vi "TALOS Root path.vi"(8 "error in (no error)":errorcluster) -> (0 "error out":errorcluster, 3 "TALOS Root Path":path)   [LabVIEW 2026, in "TALOS.lvlib"]
doc: "This VI gives the path to the root of the folder tree."
uses:
  TALOS.lvlib
  Global Memory.vi
  <vilib>/Utility/LVLibp/NI_PackedLibraryUtility.lvlib
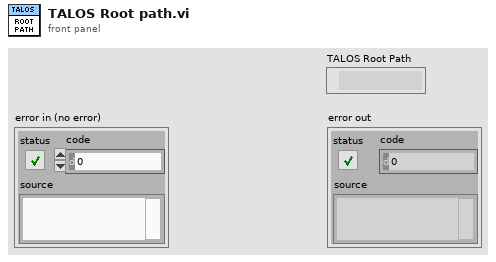
[diagram p1: front panel]
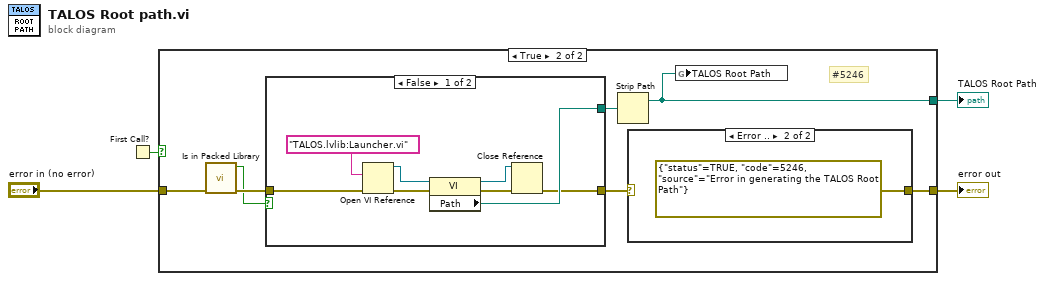
[diagram p0: block diagram]
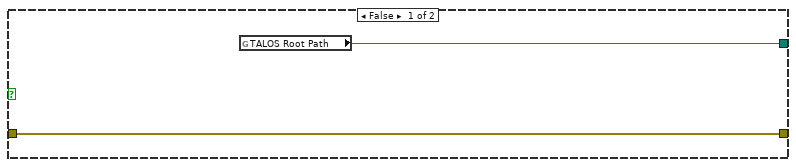
[diagram p2: hidden frame]
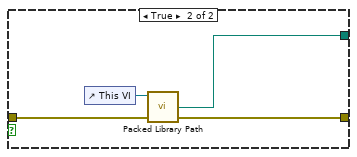
[diagram p4: hidden frame]
diagram:
  n1 = First Call?() -> (First Call?: T/F=w1:bool)
  n2 = case shown="True" w1 {
    tunnel: [w5 w12] -> w4
    tunnel: [w6 w7] -> w3
    tunnel: "error in (no error)" -> [w6 w11]
    frame False {
      n3 = global read "Global Memory.vi" "TALOS Root Path"() -> (w5:path)
    }
    frame True {
      # "#5246"
      n4 = call "Is in Packed Library.vi"("error in (no error)"=w11) -> ("error out"=w10:errorcluster, "Is In Packed Library"=w9:bool)  [unwired: 9 in]
      n5 = case shown="False" w9 {
        tunnel: w10 -> [w23 w27]
        tunnel: [w16 w24] -> w8
        tunnel: [w17 w25] -> w13
        frame False {
          n6 = Open VI Reference(vi path="TALOS.lvlib:Launcher.vi" ("string"), error in (no error)=w23) -> (vi reference=w20:refnum<vi>, error out=w21:errorcluster)  [unwired: 4 in]
          n7 = property class="VI"(reference=w20, error in=w21) -> (reference out=w18:refnum<vi>, error out=w19:errorcluster, "Path"=w17:path)
          n8 = Close Reference(reference=w18, error in (no error)=w19) -> (error out=w16:errorcluster)
        }
        frame True {
          n9 = control-ref of="This VI"() -> (w26:refnum<vi>)
          n10 = call <vilib>:"Packed Library Path.vi"("error in (no error)"=w27, "vi reference"=w26) -> ("error out"=w24:errorcluster, "packed library path"=w25:path)  [unwired: 1 in, 1 out]
        }
      }
      n11 = Strip Path(path=w13) -> (stripped path=w12:path)  [unwired: 1 out]
      n12 = case shown="Error .." w8 {
        selector: w8 -> [w14 _]
        tunnel: [w14 errorcluster {"status"=TRUE, "code"=5246, "source"="Error in generating the TALOS Root Path"} ("error IO")] -> w7
        frame No Error {
        }
        frame Error {
        }
      }
      n13 = global write "Global Memory.vi" "TALOS Root Path"(w12) -> ()
    }
  }
  "TALOS Root Path" <- w4
  "error out" <- w3
